vi "gen_tooth_function.vi"(8 "error in (no error)":errorcluster, 10 "z signal graph ref":refnum<vi>, 11 "TrajectoryAK101022Resonance in":refnum<class "TrajectoryAK101022Resonance.lvclass">) -> (0 "error out":errorcluster, 1 "z-frequency":dbl[unit], 2 "z points":dbl[unit][](array[numeric]), 3 "TrajectoryAK101022Resonance out":refnum<class "TrajectoryAK101022Resonance.lvclass">)   [LabVIEW 2010, in "TrajectoryAK101022Resonance.lvclass"]
uses:
  TrajectoryAK101022Resonance.lvclass
  FPGAWrapper/FPGAWrapperAK101022Resonance/FPGAWrapperAK101022Resonance/FPGAWrapperAK101022Resonance.lvclass
  TrajectoryAK101022Resonance.lvclass/TrajectoryAK101022Resonance.ctl
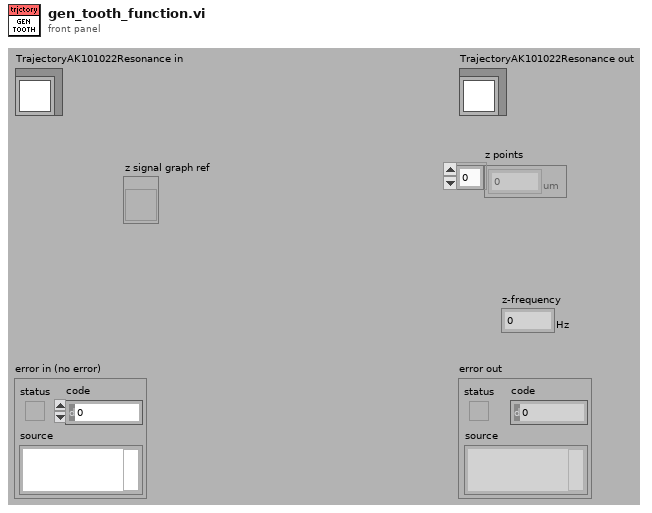
[diagram p1: front panel]
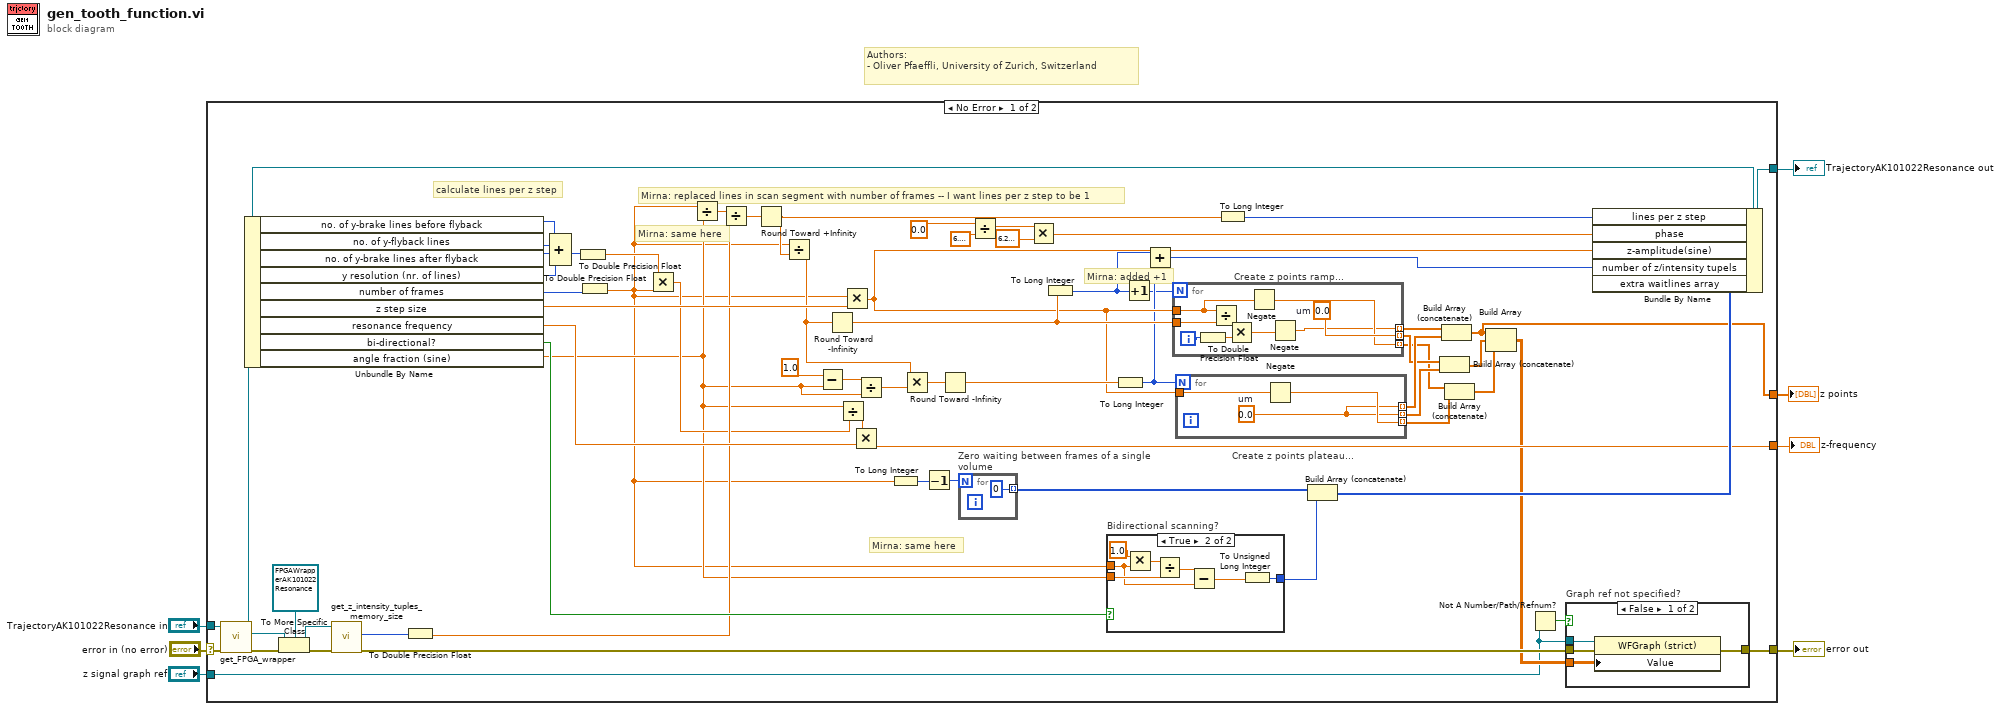
[diagram p0: block diagram]
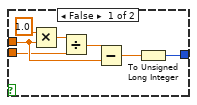
[diagram p3: hidden frame]
diagram:
  # "Authors: \n- Oliver Pfaeffli, University of Zurich, Switzerland"
  n1 = case shown="No Error" "error in (no error)" {
    selector: "error in (no error)" -> [w59 w107]
    tunnel: [w35 w107] -> w6
    tunnel: [w73 w106] -> w5
    tunnel: "TrajectoryAK101022Resonance in" -> [w58 w106]
    tunnel: [w37 _] -> w3
    tunnel: "z signal graph ref" -> [w33 _]
    tunnel: [w13 _] -> w1
    frame No Error {
      # "Mirna: same here"
      # "Mirna: added +1"
      # "Mirna: same here"
      # "Mirna: replaced lines in scan segment with number of frames -- I want lines per z step to be 1"
      # "calculate lines per z step"
      n2 = call-dynamic "get_FPGA_wrapper.vi"("error in (no error)"=w59, "TrajectoryMG100122GenericFPGA in"=w58) -> ("error out"=w55:errorcluster, "GenericFPGAWrapper.lvclass"=w56:refnum<class "GenericFPGAWrapper.lvclass">, "TrajectoryMG100122GenericFPGA out"=w57:refnum<class "TrajectoryAK101022Resonance.lvclass">)  [unwired: 7 in]
      n3 = Unbundle By Name(w57) -> ("no. of y-brake lines before flyback"=w63:i32, "no. of y-flyback lines"=w62:i32, "no. of y-brake lines after flyback"=w61:i32, "y resolution (nr. of lines)"=w43:i32, "number of frames"=w41:i32, "z step size"=w40:dbl[unit], "resonance frequency"=w44:dbl[unit], "bi-directional?"=w49:bool, "angle fraction (sine)"=w27:dbl)
      n4 = To More Specific Class(target class=refnum<class "FPGAWrapperAK101022Resonance.lvclass"> refnum ("FPGAWrapperAK101022Resonance.lvclass"), reference=w56, error in=w55) -> (specific class reference=w52:refnum<class "FPGAWrapperAK101022Resonance.lvclass">, error out=w54:errorcluster)
      n5 = call "get_z_intensity_tuples_memory_size.vi"("error in (no error)"=w54, "FPGAWrapperAK101022Resonance in"=w52) -> ("error out"=w36:errorcluster, "z/intensity memory size"=w51:i32)  [unwired: 7 in, 1 out]
      n6 = To Double Precision Float(number=w51) -> (double precision float=w39:dbl)
      n7 = Compound Arithmetic op=ADD(w63, w62, w61, w43) -> (w42:i32)
      n8 = To Double Precision Float(number=w42) -> (double precision float=w68:dbl)
      n9 = To Double Precision Float(number=w41) -> (double precision float=w8:dbl)
      n10 = Multiply(x=w68, y=w8) -> (x*y=w31:dbl)
      n11 = Divide(x=w8, y=w27) -> (x/y=w65:dbl)
      n12 = Divide(x=w65, y=w39) -> (x/y=w67:dbl)
      n13 = Round Toward +Infinity(x=w67) -> (ceil(x): smallest int >= x=w64:dbl)
      n14 = Divide(x=w8, y=w64) -> (x/y=w25:dbl)
      n15 = Subtract(x=1.0, y=w27) -> (x-y=w28:dbl)
      n16 = Round Toward -Infinity(1:w25) -> (0:w46:dbl)
      n17 = Divide(x=w27, y=w31) -> (x/y=w60:dbl)
      n18 = Multiply(x=w8, y=w40) -> (x*y=w22:dbl[unit])
      n19 = Multiply(x=w60, y=w44) -> (x*y=w37:dbl[unit])
      n20 = Divide(x=w28, y=w27) -> (x/y=w26:dbl)
      n21 = To Long Integer(number=w8) -> (32bit integer=w48:i32)
      n22 = Multiply(x=w25, y=w26) -> (x*y=w24:dbl)
      n23 = Decrement(x=w48) -> (x-1=w47:i32)
      n24 = Round Toward -Infinity(1:w24) -> (0:w23:dbl)
      n25 = for "Zero waiting between frames of a single volume" {
        N: w47 -> [_]
        tunnel: [u32 0] -> w50 mode=indexing
      }
      n26 = Divide(x=0.0, y=6.283185307179586) -> (x/y=w70:dbl)
      n27 = Multiply(x=w70, y=dbl[unit] 6.283185307179586) -> (x*y=w69:dbl[unit])
      n28 = To Long Integer(number=w46) -> (32bit integer=w12:i32)
      n29 = case "Bidirectional scanning?" shown="True" w49 {
        tunnel: w8 -> [w84 w90]
        tunnel: [w82 w95] -> w45
        tunnel: w27 -> [w83 w92]
        frame False {
          n30 = Multiply(x=1.0, y=w84) -> (x*y=w87:dbl)
          n31 = Divide(x=w87, y=w83) -> (x/y=w86:dbl)
          n32 = Subtract(x=w86, y=w84) -> (x-y=w85:dbl)
          n33 = To Unsigned Long Integer(number=w85) -> (unsigned 32bit integer=w82:u32)
        }
        frame True {
          n34 = Multiply(x=1.0, y=w90) -> (x*y=w93:dbl)
          n35 = Divide(x=w93, y=w92) -> (x/y=w91:dbl)
          n36 = Subtract(x=w91, y=w90) -> (x-y=w89:dbl)
          n37 = To Unsigned Long Integer(number=w89) -> (unsigned 32bit integer=w95:u32)
        }
      }
      n38 = To Long Integer(number=w23) -> (32bit integer=w11:i32)
      n39 = Increment(x=w12) -> (x+1=w9:i32)
      n40 = Add(x=w12, y=w11) -> (x+y=w10:i32)
      n41 = for "Create z points ramp..." {
        N: w9 -> [_]
        tunnel: w46 -> [w104]
        tunnel: w22 -> [w100]
        tunnel: [w97] -> w21 mode=indexing
        tunnel: [w101] -> w19 mode=indexing
        tunnel: [w99] -> w16 mode=indexing
        i -> [w105]
        w101 = dbl[unit] 0.0  # um
        n42 = To Double Precision Float(number=w105) -> (double precision float=w103:dbl)
        n43 = Divide(x=w100, y=w104) -> (x/y=w102:dbl[unit])
        n44 = Multiply(x=w102, y=w103) -> (x*y=w98:dbl[unit])
        n45 = Negate(x=w100) -> (-x=w99:dbl[unit])
        n46 = Negate(x=w98) -> (-x=w97:dbl[unit])
      }
      n47 = for "Create z points plateau..." {
        N: w11 -> [_]
        tunnel: w22 -> [w76]
        tunnel: [w74] -> w18 mode=indexing
        tunnel: [w75] -> w15 mode=indexing
        tunnel: [w74] -> w20 mode=indexing
        w74 = dbl[unit] 0.0  # um
        n48 = Negate(x=w76) -> (-x=w75:dbl[unit])
      }
      n49 = To Long Integer(number=w64) -> (32bit integer=w66:i32)
      n50 = Build Array (concatenate)(w50, w45) -> (w38:u32[])
      n51 = Build Array (concatenate)(w19, w18) -> (w17:dbl[unit][])
      n52 = Build Array (concatenate)(w21, w20) -> (w13:dbl[unit][])
      n53 = Build Array (concatenate)(w16, w15) -> (w14:dbl[unit][])
      n54 = Build Array(w13, w17, w14) -> (w34:dbl[unit][][])
      n55 = Not A Number/Path/Refnum?(number/path/refnum=w33) -> (NaN/Path/Refnum?=w32:bool)
      n56 = case "Graph ref not specified?" shown="False" w32 {
        tunnel: w36 -> [w80 w81]
        tunnel: [w79 w81] -> w35
        tunnel: w33 -> [w78 _]
        tunnel: w34 -> [w77 _]
        frame False {
          n57 = property class="WFGraph (strict)"(reference=w78, error in=w80, "Value"=w77) -> (error out=w79:errorcluster)  [unwired: 1 out]
        }
        frame True {
        }
      }
      n58 = Bundle By Name(cluster=w57, "lines per z step"=w66, "phase"=w69, "z-amplitude(sine)"=w22, "number of z/intensity tupels"=w10, "extra waitlines array"=w38) -> (w73:refnum<class "TrajectoryAK101022Resonance.lvclass">)
    }
    frame Error {
    }
  }
  "error out" <- w6
  "TrajectoryAK101022Resonance out" <- w5
  "z-frequency" <- w3
  "z points" <- w1
